vi "NI PXIe-411x PS RT Driver VI.vi"(6 "Device Clock":string, 9 "Device Inputs FIFO":refnum<k33>, 11 "Device Reference":T1 format="%.0x") -> ()   [LabVIEW 2023, in "NI PXIe-411x PS Custom Device.lvlib"]
uses:
  NI PXIe-411x PS Custom Device.lvlib
  <vilib>/NI VeriStand/Custom Device API/Custom Device Item Ref.ctl
  <vilib>/NI VeriStand/Custom Device API/Custom Device Channel Type.ctl
  <vilib>/Platform/TimedLoop/XDataNode/timing_clust.ctl
  <vilib>/Platform/TimedLoop/XDataNode/nitl_modes.ctl
  <vilib>/Platform/TimedLoop/XDataNode/wakeup.ctl
  411x_Global.vi
  <vilib>/NI VeriStand/Custom Device API/Get Item Property (Boolean).vi
  <vilib>/Platform/TimedLoop/XDataNode/XDataNode.xnode
  <vilib>/Platform/TimedLoop/XDataNode/XDNodeRunTimeDep.lvlib
  <vilib>/NI VeriStand/Custom Device API/Custom Device API.lvlib
  <vilib>/NI VeriStand/Custom Device Tools/Custom Device Utility Library/Custom Device Utility Library.lvlib
panel:
  in  "Status Notifier":refnum<notifier>
  # "Custom Device Template\nv1.0"
  # "Use this template as a starting point for creating a custom device code module. The input controls shown here are specially named controls that the system will use to provide the device loop with data. The controls are not required for the device loop to run. For instance, if the device doesn't produce any output data, then you don't need the Device Outputs FIFO control. If you do use these controls, however, they need to have these exact names to be functional."
  # "The optional status notifier element is used to notify the RT engine of the last state of the custom device, and to indicate the device has completed execution. If this control is not used, a default No Error value is returned to the system when the device finishes execution.\n\nNote: This error state is not checked until the system shuts down. Use an output status channel to send more immediate status values to the system."
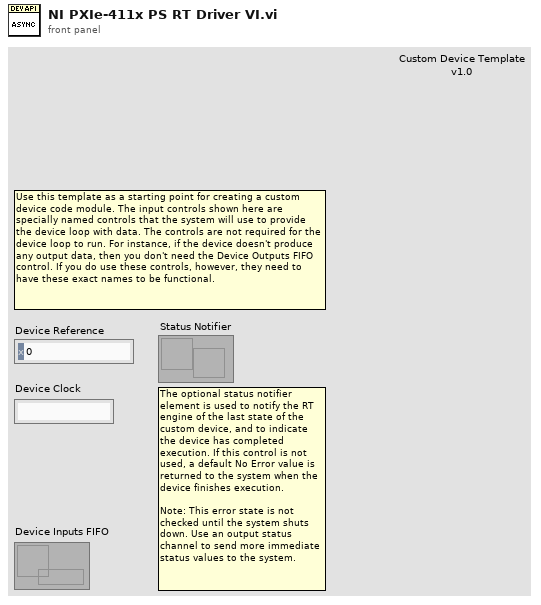
[diagram p1: front panel]
types:
  T1 = typedef "Custom Device API.lvlib/Custom Device Item Ref.ctl" = u64
  T2 = typedef "Custom Device API.lvlib/Custom Device Channel Type.ctl" = enum16{"Input", "Output"}
  T3 = typedef "Custom Device API.lvlib/Custom Device Timed Loop Priority.ctl" = enum32{"Low", "Medium", "High"}
  T4 = cluster{"instrument handle out":refnum<k15>, "Value":string, "Value":u16}[]
  T5 = typedef "XDNodeRunTimeDep.lvlib/timing_clust.ctl" = cluster{"Expected End [f-1]":u64, "Actual End [f-1]":u64, "Finished Late? [f-1]":bool, "Expected End [i-1]":u64, "Actual End [i-1]":u64, "Finished Late? [i-1]":bool, "Expected Start [i]":u64, "Actual Start [i]":u64, "Expected Start [f]":u64, "Actual Start [f]":u64, "Source Name":string, "Structure Name":string, "Period":i64, "Deadline":i64, "Offset":i64, "Start":i64, "Priority":i32, "Timeout":i32, "Mode":T6, "Wakeup Reason":T7, "Error":errorcluster, "Source Type":string, "Secondary Source Type":string, "Global End Time":u64, "Global Start Time":u64, "Frame Duration":u64, "Iteration Duration":u64, "Assigned CPU":i32, "I/O Scan Engine Mode":u32}
  T6 = typedef "XDNodeRunTimeDep.lvlib/nitl_modes.ctl" = enum32{"No Change", "Process missed periods, maintain original phase", "Discard missed periods, maintain original phase", "Process missed periods, ignore original phase", "Discard missed periods, ignore original phase"}
  T7 = typedef "XDNodeRunTimeDep.lvlib/wakeup.ctl" = enum32{"Normal", "Aborted", "Asynchronous wakeup", "Timing source error", "Timed loop error", "Timeout"}
  T8 = cluster{"V_min":dbl, "V_max":dbl, "I_min":dbl, "I_max":dbl}
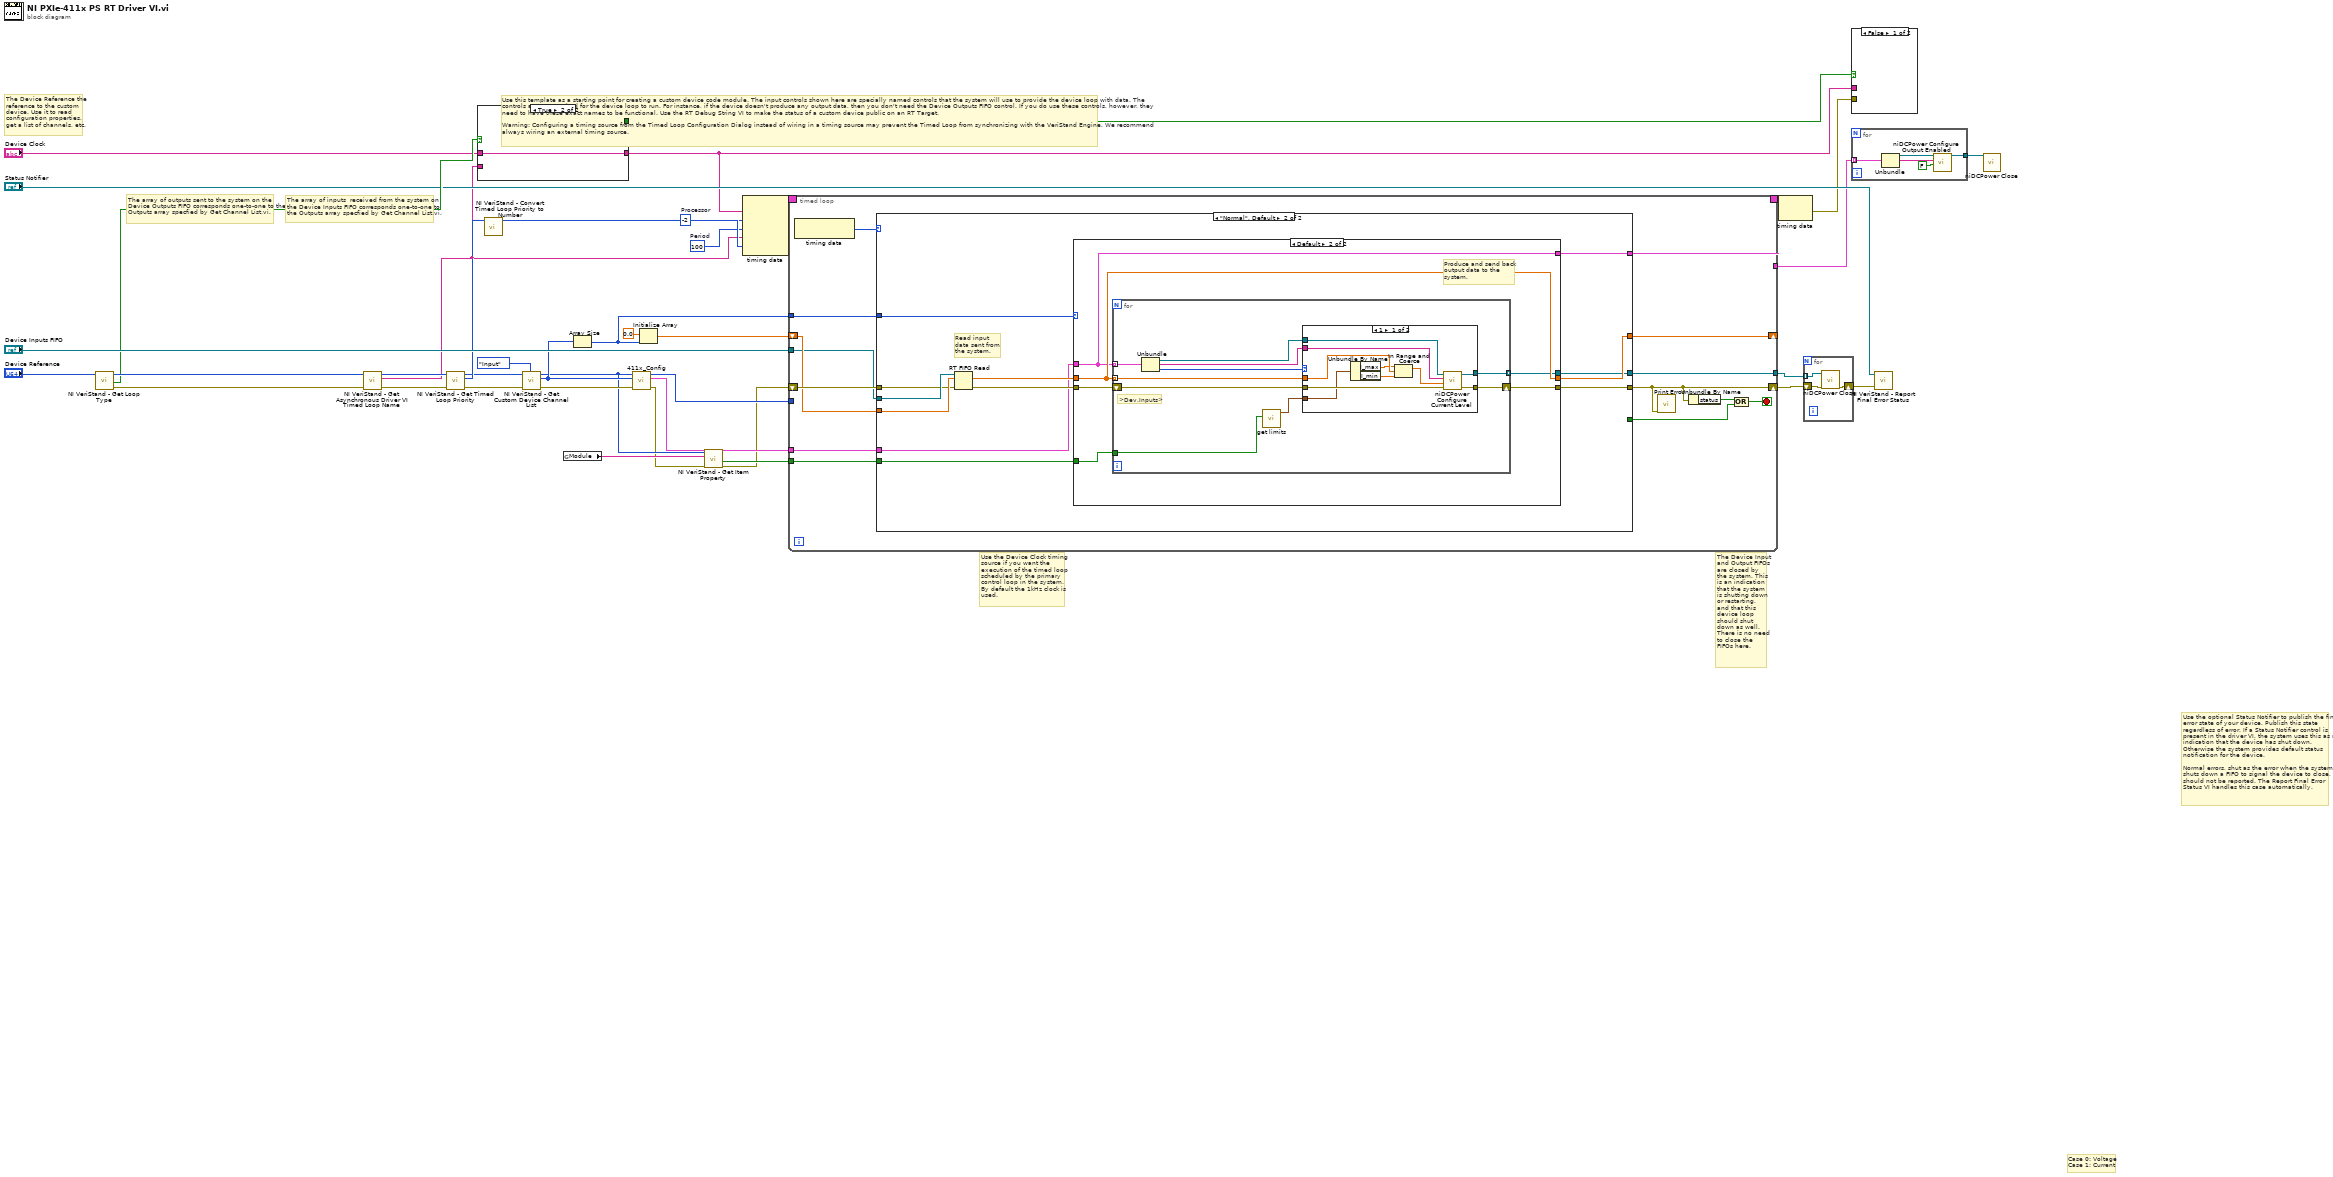
[diagram p0: block diagram]
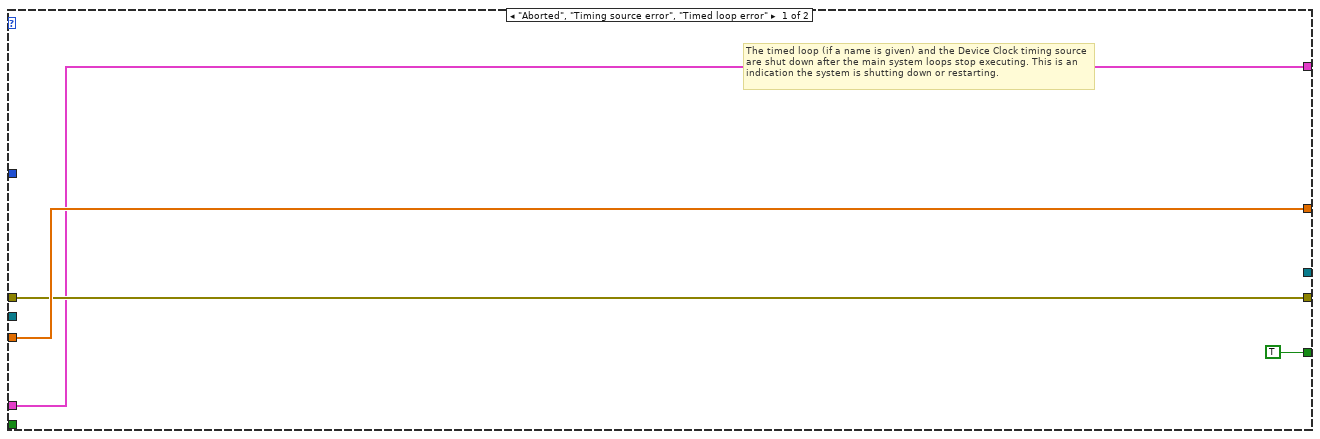
[diagram p2: hidden frame]
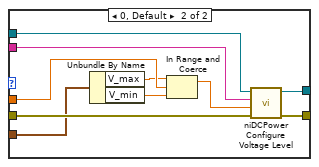
[diagram p4: hidden frame]
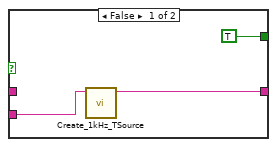
[diagram p5: hidden frame]
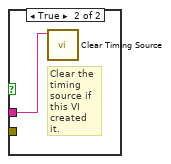
[diagram p6: hidden frame]
diagram:
  w29 = i64 100  # Period
  w30 = -2  # Processor
  # "Case 0: Voltage\nCase 1: Current"
  # "The array of inputs  received from the system on the Device Inputs FIFO corresponds one-to-one to the Outputs array specfied by Get Channel List.vi."
  # "Use the optional Status Notifier to publish the final error state of your device. Publish this state regardless of error. If a Status Notifier control is present in the driver VI, the system uses this as an indication that the device has shut down. Otherwise the system provides default status notification for the device.\n\nNormal errors, shut as the error when the system shuts down a FIFO to signal the device to close, should not be reported. The Report Final Error Status VI handles this case automatically."
  # "The Device Input and Output FIFOs are closed by the system. This is an indication that the system is shutting down or restarting, and that this device loop should shut down as well. There is no need to close the FIFOs here."
  # "The array of outputs sent to the system on the Device Outputs FIFO corresponds one-to-one to the Outputs array specfied by Get Channel List.vi."
  # "The Device Reference the reference to the custom device. Use it to read configuration properties, get a list of channels, etc."
  # "Use the Device Clock timing source if you want the execution of the timed loop scheduled by the primary control loop in the system. \nBy default the 1kHz clock is used."
  # "Use this template as a starting point for creating a custom device code module. The input controls shown here are specially named controls that the system will use to provide the device loop with data. The controls are not required for the device loop to run. For instance, if the device doesn't produce any output data, then you don't need the Device Outputs FIFO control. If you do use these controls, however, they need to have these exact names to be functional. Use the RT Debug String VI to make the status of a custom device public on an RT Target.\n\nWarning: Configuring a timing source from the Timed Loop Configuration Dialog instead of wiring in a timing source may prevent the Timed Loop from synchronizing with the VeriStand Engine. We recommend always wiring an external timing source."
  n1 = call <vilib>:"NI VeriStand - Get Loop Type.vi"("Device Ref in"="Device Reference") -> ("error out"=w28:errorcluster, "Use Device Clock"=w25:bool, "Device Ref out"=w27:T1)  [unwired: 1 in, 7 out]
  n2 = call <vilib>:"NI VeriStand - Get Asynchronous Driver VI Timed Loop Name.vi"("error in (no error)"=w28, "Device Ref in"=w27) -> ("error out"=w33:errorcluster, "Device Timed Loop Name"=w19:string, "Device Ref out"=w39:T1)  [unwired: 7 out]
  n3 = call <vilib>:"NI VeriStand - Get Timed Loop Priority.vi"("error in (no error)"=w33, "Device Ref in"=w39) -> ("error out"=w9:errorcluster, "Priority"=w32:T3, "Device Ref out"=w18:T1)  [unwired: 7 out]
  n4 = case shown="True" w25 {
    tunnel: "Device Clock" -> [_ w43]
    tunnel: [w42 w43] -> w20
    tunnel: [TRUE _] -> w21
    tunnel: w19 -> [w40 _]
    frame False {
      n5 = call <vilib>:"Create_1kHz_TSource.vi"("name (in)"=w40) -> ("name (out)"=w42:string)  [unwired: 1 in, 9 out]
    }
    frame True {
    }
  }
  n6 = call <vilib>:"NI VeriStand - Convert Timed Loop Priority to Number.vi"("Priority"=w32) -> ("Numeric Priority"=w31:i32)  [unwired: 10 out]
  n7 = call <vilib>:"NI VeriStand - Get Custom Device Channel List.vi"("Channel Type"=Custom_Device_Channel_Type."Input", "error in (no error)"=w9, "Device Ref in"=w18) -> ("error out"=w15:errorcluster, "Specified Channel Ref List"=w16:T1[], "Device Ref out"=w7:T1)  [unwired: 6 out]
  n8 = global read "411x_Global.vi" "Module"() -> (w8:string)
  n9 = Array Size(array=w16) -> (size(s)=w10:i32)
  n10 = call "411x_Config.vi"("error in (no error)"=w15, "Specified Channel Ref List"=w16, "Device Ref out"=w7) -> ("error out"=w2:errorcluster, "Channel Info"=w14:T4, "Channel Ref List (out)"=w17:T1[])  [unwired: 6 in]
  n11 = Initialize Array(0.0 ("element"), w10) -> (w34:dbl[])
  n12 = call-poly <vilib>:"NI VeriStand - Get Item Property.vi"("error in (no error)"=w2, "Property Name"=w8, "Item Ref in"=w7) -> ("error out"=w1:errorcluster, "Value"=w6:bool)  [unwired: 5 in, 2 out]
  n13 = node-c288(w20, w30, w29, w19, w31) -> (w37:T5)
  n14 = timed-loop {
    timing: w37 -> [_]
    timing-out: [_] -> w36
    shift-right: [w55] -> _
    shift-left: w34 -> [w56]
    shift-right: [w46] -> w5
    shift-left: w1 -> [w57]
    tunnel: "Device Inputs FIFO" -> [w53]
    tunnel: w10 -> [w49]
    tunnel: w17 -> [_]
    tunnel: w14 -> [w48]
    tunnel: [w47] -> w13
    tunnel: w6 -> [w45]
    tunnel: [w44] -> w3
    stop <- w50 stop-if-true
    n15 = node-c288() -> (w54:T7)  [unwired: 1 out]
    n16 = case shown="\"Normal\", Default" w54 {
      tunnel: w57 -> [w62 w70]
      tunnel: w56 -> [w63 w74]
      tunnel: [w62 w71] -> w46
      tunnel: [w63 w69] -> w55
      tunnel: w53 -> [_ w75]
      tunnel: [TRUE _] -> w51
      tunnel: w49 -> [_ w68]
      tunnel: w48 -> [w60 w67]
      tunnel: [w60 w66] -> w47
      tunnel: w45 -> [_ w65]
      tunnel: [_ w64] -> w44
      frame "Aborted", "Timing source error", "Timed loop error" {
        # "The timed loop (if a name is given) and the Device Clock timing source are shut down after the main system loops stop executing. This is an indication the system is shutting down or restarting."
      }
      frame "Normal", Default {
        # "Read input data sent from the system."
        n17 = RT FIFO Read(0:w75, 1:w74, 3:w70) -> (9:w73:dbl[], 11:w72:errorcluster)  [unwired: 4 out]
        n18 = case shown="Default" w68 {
          tunnel: w73 -> [w78 w84]
          tunnel: w72 -> [w77 w83]
          tunnel: [w77 w82] -> w71
          tunnel: [w78 w84] -> w69
          tunnel: w67 -> [w76 w81]
          tunnel: [w76 w81] -> w66
          tunnel: w65 -> [_ w80]
          tunnel: [_ w79] -> w64
          frame 0 {
            # "No outputs to write to system. The Device Outputs FIFO is never created in this case, so don't write to it."
          }
          frame Default {
            # "Produce and send back output data to the system."
            n19 = for {
              tunnel: w81 -> [w94] mode=indexing
              tunnel: w84 -> [w89] mode=indexing
              shift-right: [w91] -> w82
              shift-left: w83 -> [w92]
              tunnel: w80 -> [w86]
              tunnel: [w85] -> w79 mode=indexing
              # ">Dev.Inputs>"
              n20 = Unbundle(w94) -> ("instrument handle out"=w93:refnum<k15>, "Value"=w88:string, "Value"=w90:u16)
              n21 = call "get limits.vi"("4112?"=w86) -> ("output cluster"=w87:T8)  [unwired: 10 in]
              n22 = case shown="1" w90 {
                tunnel: w93 -> [w104 w114]
                tunnel: w88 -> [w102 w112]
                tunnel: w89 -> [w101 w111]
                tunnel: w92 -> [w103 w113]
                tunnel: [w96 w106] -> w91
                tunnel: w87 -> [w99 w109]
                tunnel: [w95 w105] -> w85
                frame 1 {
                  n23 = Unbundle By Name(w99) -> ("I_max"=w98:dbl, "I_min"=w97:dbl)
                  n24 = In Range and Coerce(upper limit=w98, x=w101, lower limit=w97) -> (coerced(x)=w100:dbl)  [unwired: 1 out]
                  n25 = call <instrlib>:"niDCPower Configure Current Level.vi"("error in (no error)"=w103, "current level"=w100, "channel name"=w102, "instrument handle"=w104) -> ("error out"=w96:errorcluster, "instrument handle out"=w95:refnum<k15>)  [unwired: 6 in]
                }
                frame 0, Default {
                  n26 = Unbundle By Name(w109) -> ("V_max"=w108:dbl, "V_min"=w107:dbl)
                  n27 = In Range and Coerce(upper limit=w108, x=w111, lower limit=w107) -> (coerced(x)=w110:dbl)  [unwired: 1 out]
                  n28 = call <instrlib>:"niDCPower Configure Voltage Level.vi"("error in (no error)"=w113, "voltage level"=w110, "channel name"=w112, "instrument handle"=w114) -> ("error out"=w106:errorcluster, "instrument handle out"=w105:refnum<k15>)  [unwired: 6 in]
                }
              }
            }
          }
        }
      }
    }
    n29 = call "Print Error.vi"("error out"=w46) -> ()  [unwired: 10 in]
    n30 = Unbundle By Name(w46) -> ("status"=w52:bool)
    n31 = Compound Arithmetic op=OR(w52, w51) -> (w50:bool)
  }
  n32 = node-c288(w36) -> (w22:errorcluster)
  n33 = for {
    shift-right: [w117] -> w4
    shift-left: w5 -> [w118]
    tunnel: w3 -> [w116] mode=indexing
    n34 = call <instrlib>:"niDCPower Close.vi"("error in (no error)"=w118, "instrument handle"=w116) -> ("error out"=w117:errorcluster)  [unwired: 9 in]
  }
  n35 = case shown="False" w21 {
    tunnel: w22 -> [_ _]
    tunnel: w20 -> [_ w119]
    frame False {
    }
    frame True {
      # "Clear the timing source if this VI created it."
      n36 = call <vilib>:"Clear Timing Source.vi"("name"=w119) -> ()  [unwired: 1 in, 10 out]
    }
  }
  n37 = for {
    tunnel: w13 -> [w124] mode=indexing
    tunnel: [w120] -> w11
    n38 = Unbundle(w124) -> ("instrument handle out"=w123:refnum<k15>, "Value"=w122:string)  [unwired: 1 out]
    n39 = call <instrlib>:"niDCPower Configure Output Enabled.vi"("output enabled"=FALSE, "channel name"=w122, "instrument handle"=w123) -> ("instrument handle out"=w120:refnum<k15>)  [unwired: 7 in, 1 out]
  }
  n40 = call <vilib>:"NI VeriStand - Report Final Error Status.vi"("error in (no error)"=w4, "Status Notifier"="Status Notifier") -> ()  [unwired: 1 in, 9 out]
  n41 = call <instrlib>:"niDCPower Close.vi"("instrument handle"=w11) -> ()  [unwired: 10 in, 1 out]
